vi "例6-19.vi"() -> ()   [LabVIEW 2019]
uses:
  <vilib>/Analysis/NI_AALPro.lvlib
panel:
  out "残差":dbl format="%#_3g"
  out "斜率":dbl format="%#_4g"
  out "截距":dbl format="%#_3g"
  out "XY图":cluster{"Xi":dbl[], "Best Linear Fit":dbl[]}[](graph)
  out "拟合值":dbl[](array[numeric]) format="%_3g"
  in  "Yi":dbl[](array[numeric])
  in  "Xi":dbl[](array[numeric])
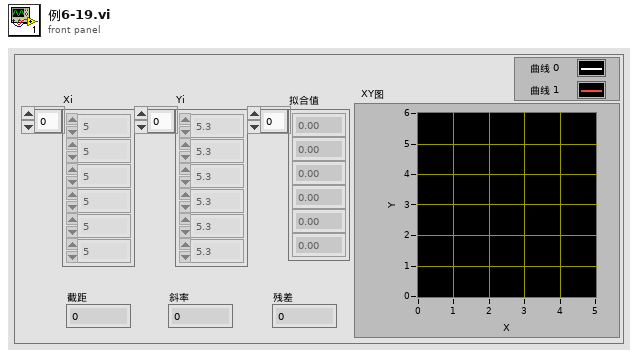
[diagram p1: front panel]
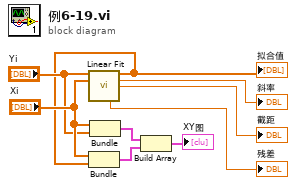
[diagram p0: block diagram]
diagram:
  n1 = call <vilib>:"Linear Fit.vi"("Y"="Yi", "X"="Xi") -> ("Best Linear Fit"=w7:dbl[], "slope"=→"斜率":dbl, "intercept"=→"截距":dbl, "residue"=→"残差":dbl)  [unwired: 9 in, 1 out]
  "拟合值" <- w7
  n2 = Bundle("Xi"="Xi", "Best Linear Fit"=w7) -> (w5:cluster{"Xi":dbl[], "Best Linear Fit":dbl[]})  [unwired: 1 in]
  n3 = Bundle("Xi"="Xi", "Yi"="Yi") -> (w6:cluster{"Xi":dbl[], "Yi":dbl[]})  [unwired: 1 in]
  n4 = Build Array(w6, w5) -> (→"XY图":cluster{"Xi":dbl[], "Best Linear Fit":dbl[]}[])
